vi "Read.vi"(8 "error in (no error)":errorcluster, 11 "Double Float.lvclass in":refnum<class "DAQmx-Bus_Waveform_Type.lvclass">) -> (0 "error out":errorcluster, 2 "Waveform":waveform(dbl), 3 "Double Float.lvclass out":refnum<class "DAQmx-Bus_Waveform_Type.lvclass">)   [LabVIEW 2021, in "DAQmx-Bus_Waveform_Type.lvclass"]
doc: "Abstract Data Classes 2.1.1.13\nTim Streeter - TSA\nCopyright (c) 2025, TSA"
uses:
  DAQmx-Bus_Waveform_Type.lvclass
  DAQmx-Bus_Waveform_Type.lvclass/DAQmx-Bus_Waveform_Type.ctl
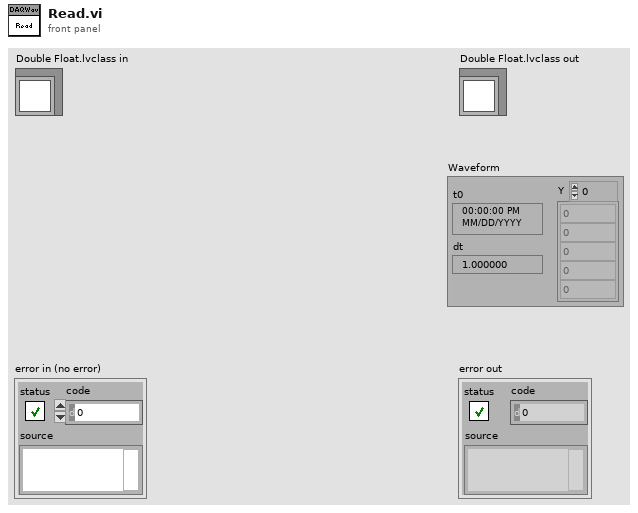
[diagram p1: front panel]
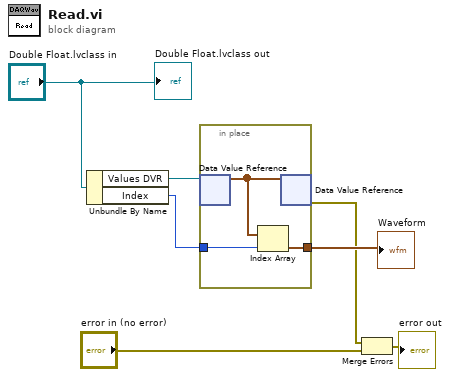
[diagram p0: block diagram]
diagram:
  n1 = Unbundle By Name("Double Float.lvclass in") -> ("Values DVR"=w6:refnum<data-value>, "Index"=w5:i32)
  n2 = in-place {
    in-place-border: w5 -> [w9]
    in-place-border: [w8] -> w4
    n3 = in-place-dvr #1(w6) -> (w10:waveform(dbl)[])  [unwired: 1 out]
    n4 = Index Array(array=w10, index=w9) -> (element=w8:waveform(dbl))
    n5 = in-place-dvr #1(w10) -> (w1:errorcluster)  [unwired: 1 out]
  }
  "Waveform" <- w4
  n6 = Merge Errors(w1, "error in (no error)") -> (→"error out":errorcluster)
  "Double Float.lvclass out" <- "Double Float.lvclass in"
